vi "LV to ITX XY2 AutoPlot.vi"(8 "error in":errorcluster, 9 "Notes":string, 10 "Data (Dictionary)":T1[](array[typedef]), 11 "path":path=path "C:/") -> (0 "error out":errorcluster, 3 "file out":path)   [LabVIEW 2016, in "LV-Data.ITX.lvclass"]
doc: "Write data to ITX file. This AutoPlot VI adds commands to automatically create a graph in Igor to quickly view your data.\n\n-- path: base path to save data\n-- filename: base filename\n-- Notes: add any notes here to help you remember what experiment you did\n-- Data: Cluster array\n It is recommended that you make the first cluster an array of timestamps\n-- wavenames: Give each data array a unique name such as \"time, bias, current,...\"zz\n-- X,Y Labels: For plotting in Igor. Can be ignored.\n-- X,Y Log: Do you wan to show X or Y on Log scale in Igor?"
uses:
  LV-Data.ITX.lvclass
  LV-Data/Typedefs/Dictionary--cluster.ctl
  C:/Users/patrick/Documents/GitHub/LV-to-ITX/src/LV-Data/LV-Data.lvclass
  LV-Data/Typedefs/Operation--enum.ctl
  LV-Data/LV-Data.lvclass/LV-Data.ctl
  LV-Data/LV-Data.lvclass
panel:
  in  "X,Y Log":i32[](array[numeric])
  in  "X,Y Labels":string[](array[string])=["x label", "y label"]
  # "Below are relevant for creating graphs in Igor"
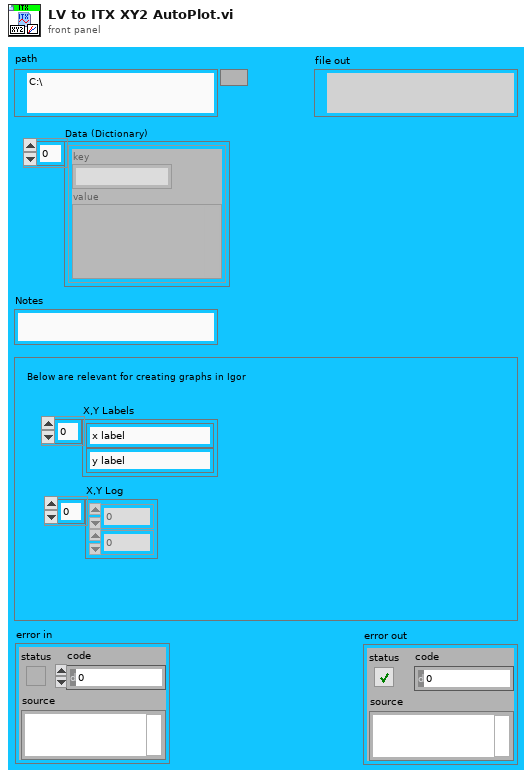
[diagram p1: front panel]
types:
  T1 = typedef "LV-Data.lvclass/Dictionary--cluster.ctl" = cluster{"key":string, "value":variant}
  T2 = typedef "LV-Data.lvclass/Operation--enum.ctl" = enum16{"Read", "Write", "Write + Append"}
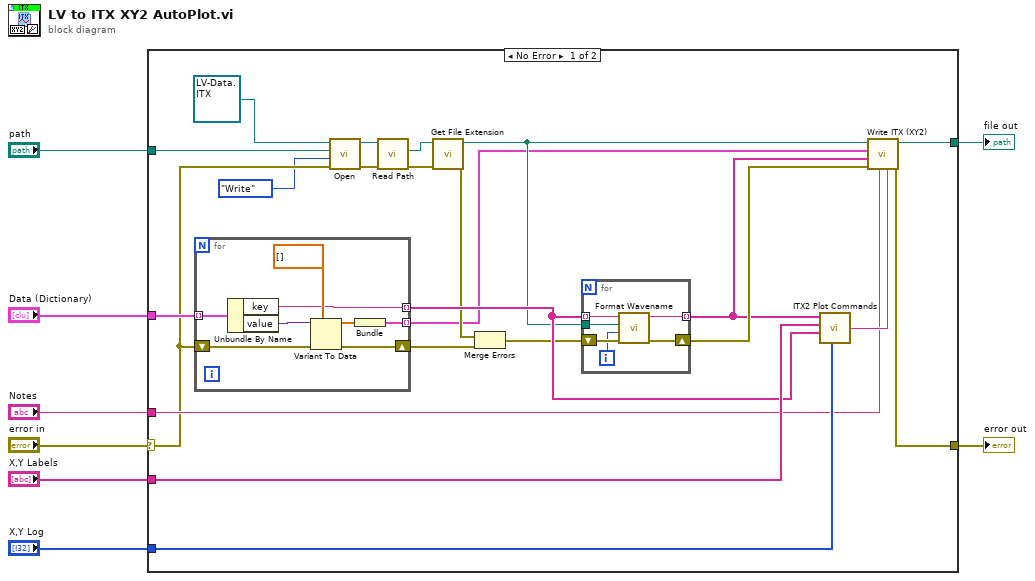
[diagram p0: block diagram]
diagram:
  n1 = case shown="No Error" "error in" {
    selector: "error in" -> [w13 w47]
    tunnel: "path" -> [w9 w46]
    tunnel: "X,Y Labels" -> [w31 _]
    tunnel: [w30 w46] -> w6
    tunnel: "X,Y Log" -> [w29 _]
    tunnel: [w24 w47] -> w4
    tunnel: "Data (Dictionary)" -> [w28 _]
    tunnel: "Notes" -> [w15 _]
    frame No Error {
      n2 = for {
        tunnel: w28 -> [w39] mode=indexing
        tunnel: [w33] -> w17 mode=indexing
        shift-right: [w34] -> w21
        shift-left: w13 -> [w37]
        tunnel: [w32] -> w27 mode=indexing
        n3 = Unbundle By Name(w39) -> ("key"=w32:string, "value"=w38:variant)
        n4 = Variant To Data(error in=w37, type=dbl[] [], Variant=w38) -> (data=w35:dbl[], error out=w34:errorcluster)
        n5 = Bundle(w35) -> (w33:cluster{dbl[]})  [unwired: 1 in]
      }
      n6 = call-dynamic "Open.vi"("error in (no error)"=w13, "Operation"=Operation--enum."Write", "Path"=w9, "Data in"=refnum<class "LV-Data.ITX.lvclass"> refnum ("Data.ITX.lvclass")) -> ("error out"=w12:errorcluster, "Data out"=w11:refnum<class "LV-Data.ITX.lvclass">)  [unwired: 6 in]
      n7 = call "Read Path.vi"("error in (no error)"=w12, "Data Save"=w11) -> ("error out"=w22:errorcluster, "Path"=w23:path)  [unwired: 7 in, 1 out]
      n8 = call <vilib>:"Get File Extension.vi"("error in (no error)"=w22, "file"=w23) -> ("error out"=w20:errorcluster, "dup file"=w18:path)  [unwired: 5 in, 3 out]
      n9 = Merge Errors(w20, w21) -> (w19:errorcluster)
      n10 = for {
        tunnel: w27 -> [w45] mode=indexing
        shift-right: [w43] -> w25
        shift-left: w19 -> [w44]
        tunnel: [w42] -> w16 mode=indexing
        tunnel: w18 -> [w40]
        i -> [w41]
        n11 = call "Format Wavename.vi"("error in (no error)"=w44, "Index"=w41, "Path"=w40, "Name"=w45) -> ("error out"=w43:errorcluster, "Formatted wavename"=w42:string)  [unwired: 6 in]
      }
      n12 = call "ITX2 Plot Commands.vi"("X,Y Log"=w29, "Plot labels"=w27, "X,Y Labels"=w31, "wavenames"=w16) -> ("result string"=w26:string)  [unwired: 2 in]
      n13 = call "Write ITX (XY2).vi"("Commands"=w26, "Notes"=w15, "error in"=w25, "Wavenames"=w16, "array of clusters"=w17, "filename"=w18) -> ("error out"=w24:errorcluster, "file"=w30:path)  [unwired: 4 in]
    }
    frame Error {
    }
  }
  "file out" <- w6
  "error out" <- w4
